vi "Find_Missing_Serial_Ports.vi"(1 "Serial Port Aliases":string[][](array[string]), 2 "Must have Port?":bool, 3 "Aliase to Check":string) -> (0 "Serial Port Aliases Out":string[][](array[string]))   [LabVIEW 2022 SP3]
uses:
  <vilib>/Instr/_visa.llb/VISA Find Search Mode.ctl
  Anemometry/Anemometry Sub Vis/Globals/Constants_global.vi
  Anemometry/Anemometry Sub Vis/Globals/Meas_global.vi
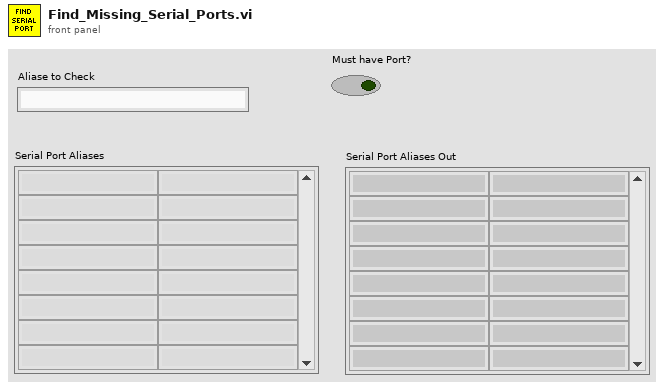
[diagram p1: front panel]
types:
  T1 = typedef "VISA Find Search Mode.ctl" = u32
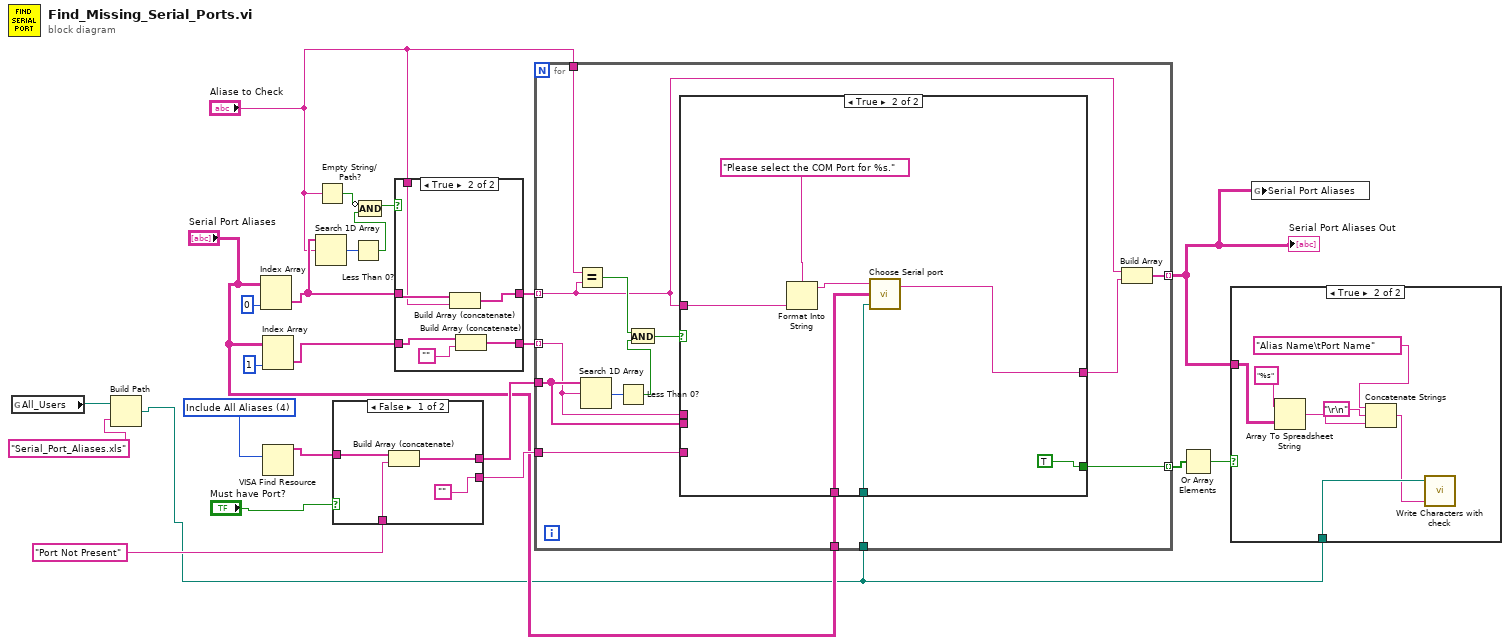
[diagram p0: block diagram]
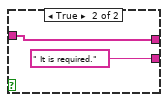
[diagram p2: hidden frame]
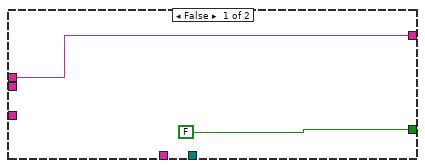
[diagram p5: hidden frame]
diagram:
  w19 = T1 4 items=["Canonical Names Only"=0, "Aliases Only"=1, "Include Matching Aliases"=2, "Include All Aliases"=4] ("Search Mode")
  n1 = global read "Constants_global.vi" "All_Users"() -> (w24:path)
  n2 = Build Path(base path=w24, name or relative path="Serial_Port_Aliases.xls") -> (appended path=w1:path)
  n3 = Index Array(array="Serial Port Aliases", index (col)=0 ("disabled index (col)")) -> (element=w16:string[])  [unwired: 1 in]
  n4 = Index Array(array="Serial Port Aliases", index (col)=1 ("disabled index (col)")) -> (element=w14:string[])  [unwired: 1 in]
  n5 = VISA Find Resource(10:w19) -> (3:w7:string[])  [unwired: 2 in, 2 out]
  n6 = Search 1D Array(1D array=w16, element="Aliase to Check") -> (index of element=w12:i32)  [unwired: 1 in]
  n7 = Empty String/Path?(string/path="Aliase to Check") -> (empty?=w8:bool)
  n8 = case shown="False" "Must have Port?" {
    tunnel: w7 -> [w28 w30]
    tunnel: [w27 w30] -> w6
    tunnel: ["" " It is required."] -> w4
    tunnel: "Port Not Present" -> [w25 _]
    frame False {
      n9 = Build Array (concatenate)(w28, w25) -> (w27:string[])
    }
    frame True {
    }
  }
  n10 = Less Than 0?(x=w12) -> (x < 0?=w9:bool)
  n11 = Compound Arithmetic op=AND(invert w8, w9) -> (w10:bool)
  n12 = case shown="True" w10 {
    tunnel: w16 -> [w32 w38]
    tunnel: [w32 w37] -> w15
    tunnel: w14 -> [w31 w34]
    tunnel: [w31 w35] -> w13
    tunnel: "Aliase to Check" -> [_ w36]
    frame False {
    }
    frame True {
      n13 = Build Array (concatenate)(w38, w36) -> (w37:string[])
      n14 = Build Array (concatenate)(w34, "") -> (w35:string[])
    }
  }
  n15 = for {
    tunnel: w6 -> [w52]
    tunnel: w13 -> [w51] mode=indexing
    tunnel: w15 -> [w43] mode=indexing
    tunnel: [w50] -> w3 mode=indexing
    tunnel: [w44] -> w18 mode=indexing
    tunnel: "Aliase to Check" -> [w48]
    tunnel: w4 -> [w41]
    tunnel: "Serial Port Aliases" -> [w40]
    tunnel: w1 -> [w39]
    n16 = Equal?(x=w48, y=w43) -> (x = y?=w46:bool)
    n17 = Search 1D Array(1D array=w52, element=w51) -> (index of element=w49:i32)  [unwired: 1 in]
    n18 = Less Than 0?(x=w49) -> (x < 0?=w47:bool)
    n19 = And(x=w46, y=w47) -> (x .and. y?=w45:bool)
    n20 = case shown="True" w45 {
      tunnel: w52 -> [_ _]
      tunnel: w43 -> [_ w60]
      tunnel: [w54 w58] -> w42
      tunnel: w51 -> [w54 _]
      tunnel: [FALSE TRUE] -> w44
      tunnel: w41 -> [_ _]
      tunnel: w40 -> [_ w56]
      tunnel: w39 -> [_ w55]
      frame False {
      }
      frame True {
        n21 = Format Into String(format string="Please select the COM Port for %s." ("Message"), w60) -> (resulting string=w59:string)  [unwired: 2 in, 1 out]
        n22 = call "Choose Serial port.vi"("Path"=w55, "Current Serial Port Aliases"=w56, "Message"=w59) -> ("Choosen Port"=w58:string)  [unwired: 1 in]
      }
    }
    n23 = Build Array(w43, w42) -> (w50:string[])
  }
  "Serial Port Aliases Out" <- w3
  n24 = Or Array Elements(Boolean array=w18) -> (logical OR=w17:bool)
  n25 = case shown="True" w17 {
    tunnel: w3 -> [_ w67]
    tunnel: w1 -> [_ w63]
    frame False {
    }
    frame True {
      n26 = Array To Spreadsheet String(array=w67, 3:"%s" ("format string")) -> (spreadsheet string=w66:string)  [unwired: 1 in]
      n27 = Concatenate Strings("Alias Name\tPort Name", "\r\n", w66) -> (w62:string)
      n28 = call "Write Characters with check.vi"("String to Write"=w62, "file (use dialog)"=w63) -> ()  [unwired: 2 in, 1 out]
    }
  }
  n29 = global write "Meas_global.vi" "Serial Port Aliases"(w3) -> ()
